vi "Get DDG External Output Polarity.vi"(8 "error in (no error)":errorcluster, 10 "puiPolarity":u32, 11 "uiIndex":u32) -> (0 "error out":errorcluster, 2 "puiPolarity out":u32, 3 "function return":u32)   [LabVIEW 2014, in "atmcd32d.lvlib"]
doc: "unsigned int WINAPI GetDDGExternalOutputPolarity(at_u32 uiIndex, at_u32 * puiPolarity);"
uses:
  atmcd32d.lvlib
  atmcd32d.dll
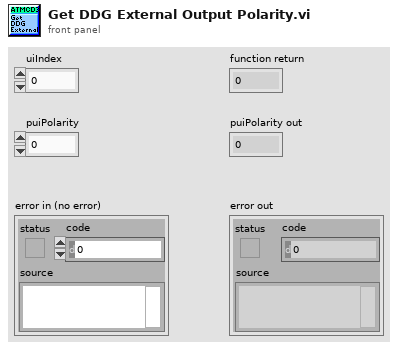
[diagram p1: front panel]
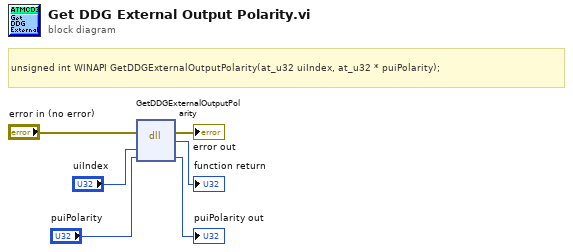
[diagram p0: block diagram]
diagram:
  # "unsigned int WINAPI GetDDGExternalOutputPolarity(at_u32 uiIndex, at_u32 * puiPolarity);"
  n1 = dll-call lib="C:/Users/Bakir/Documents/Lambda2-Testing/lib/Andorlib/atmcd32d.*" fn="GetDDGExternalOutputPolarity"(error in="error in (no error)", "uiIndex"="uiIndex", "puiPolarity"="puiPolarity") -> (error out=→"error out":errorcluster, →"function return":u32, "puiPolarity"=→"puiPolarity out":u32)  [unwired: 3 in, 1 out]
